vi "Read_write_Variant.vi"(4 "Vriant IN":variant) -> (1 "Variant out":variant, 2 "Select ?":bool=TRUE)   [LabVIEW 2015]
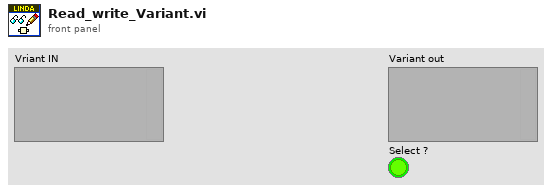
[diagram p1: front panel]
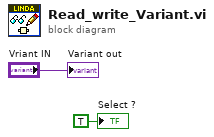
[diagram p0: block diagram]
diagram:
  "Variant out" <- "Vriant IN"
  "Select ?" <- TRUE
